vi "TSM SSC DAQmx Write (Digital Bool) Broadcast.vi"(0 "DAQ TSM in":T1, 1 "auto start(T)":bool=TRUE, 5 "Static State In":bool, 11 "error in":errorcluster) -> (4 "DAQ TSM Out":T1, 15 "error out":errorcluster)   [LabVIEW 2020]
doc: "Writes Static Digital State to a task that contains one or more digital output channels for all sites."
uses:
  Pin Map/TSM DAQmx Multi-Task.ctl
  <vilib>/NI_TestStand_SemiconductorModule/NI_TestStand_Semiconductor_Module.lvlibp/PinMap/PinQueryContext/MultiplePinMultipleSessionQueryContext/MultiplePinMultipleSessionQueryContext.lvclass
  Pin Map/SSC DAQmx.ctl
  <vilib>/DAQmx/write.llb/DAQmx Write (Digital 1D Bool NChan 1Samp 1Line).vi
  <vilib>/DAQmx/miscellaneous.llb/DAQmx Fill In Error Info.vi
  <resource>/objmgr/daqmx.rc
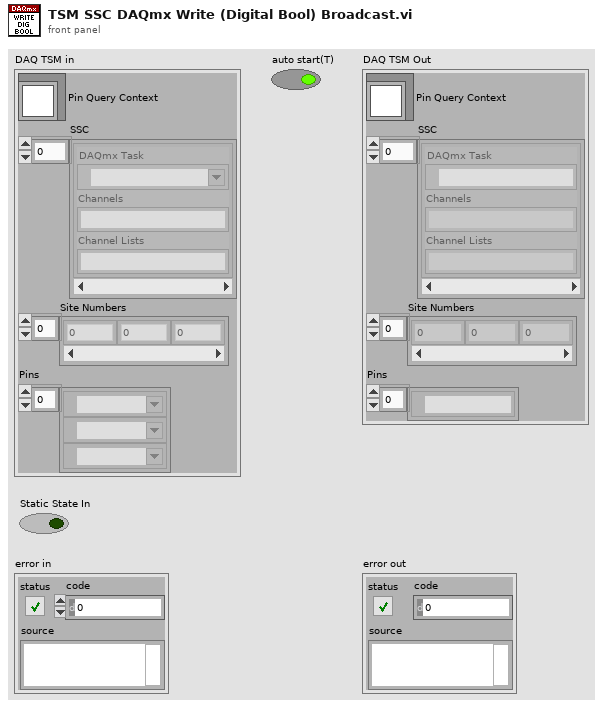
[diagram p1: front panel]
types:
  T1 = typedef "TSM DAQmx Multi-Task.ctl" = cluster{"Pin Query Context":refnum<class "MultiplePinMultipleSessionQueryContext.lvclass">, "SSC":T2[], "Site Numbers":i32[], "Pins":tag[]}
  T2 = typedef "SSC DAQmx.ctl" = cluster{"DAQmx Task ":refnum<k21>, "Channels":string, "Channel Lists":string}
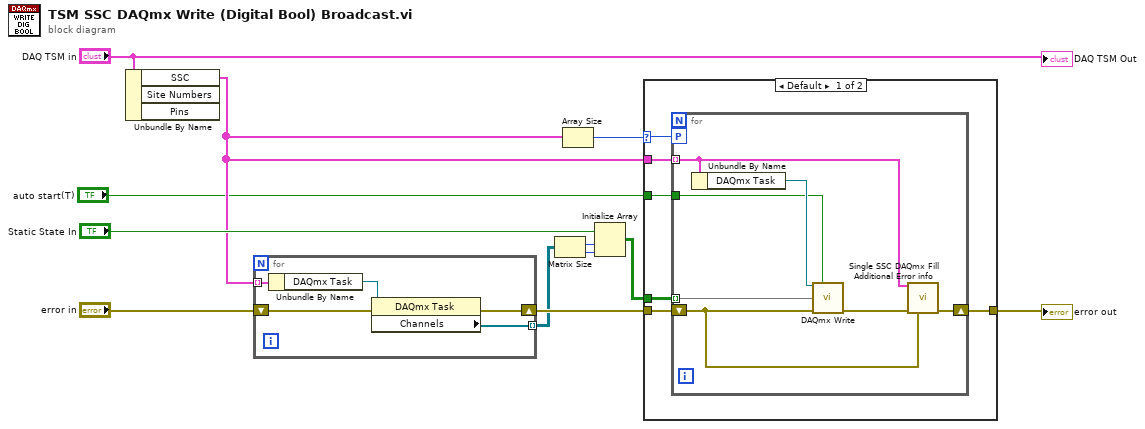
[diagram p0: block diagram]
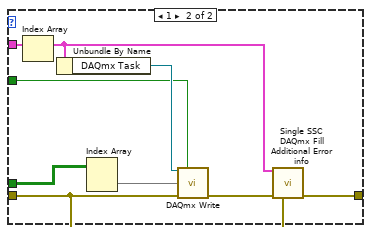
[diagram p2: hidden frame]
diagram:
  n1 = Unbundle By Name("DAQ TSM in") -> ("SSC"=w2:T2[])  [unwired: 2 out]
  n2 = for {
    shift-right: [w16] -> w8
    shift-left: "error in" -> [w17]
    tunnel: [w14] -> w5 mode=indexing
    tunnel: w2 -> [w13] mode=indexing
    n3 = Unbundle By Name(w13) -> ("DAQmx Task"=w15:refnum<k21>)
    n4 = property class="DAQmx Task"(reference=w15, error in=w17) -> (error out=w16:errorcluster, "Channels"=w14:refnum<k21>[])  [unwired: 1 out]
  }
  n5 = Matrix Size(0:w5) -> (1:w4:i32, 2:w3:i32)
  n6 = Array Size(array=w2) -> (size(s)=w9:i32)
  n7 = Initialize Array("Static State In", w4, w3) -> (w6:bool[][])
  n8 = case shown="Default" w9 {
    selector: w9 -> [w21 _]
    tunnel: [w23 w39] -> w10
    tunnel: w8 -> [w22 w38]
    tunnel: w2 -> [w20 w37]
    tunnel: w6 -> [w19 w33]
    tunnel: "auto start(T)" -> [w18 w31]
    frame Default {
      n9 = for {
        tunnel: w20 -> [w27] mode=indexing
        workers-P: w21 -> [_]
        shift-right: [w30] -> w23
        shift-left: w22 -> [w29]
        tunnel: w19 -> [w25] mode=indexing
        tunnel: w18 -> [w24]
        n10 = Unbundle By Name(w27) -> ("DAQmx Task"=w26:refnum<k21>)
        n11 = call-poly <vilib>:"DAQmx Write.vi"("task/channels in"=w26, "auto start"=w24, "data"=w25, "error in"=w29) -> ("error out"=w28:errorcluster)  [unwired: 9 in, 2 out]
        n12 = call "Single SSC DAQmx Fill Additional Error info.vi"("DAQmx SSC in"=w27, "error in"=w28, "previous error in"=w29) -> ("error out"=w30:errorcluster)  [unwired: 12 in]
      }
    }
    frame 1 {
      n13 = Index Array(array=w37) -> (element=w34:T2)  [unwired: 1 in]
      n14 = Unbundle By Name(w34) -> ("DAQmx Task"=w35:refnum<k21>)
      n15 = Index Array(array=w33) -> (element=w32:bool[])  [unwired: 2 in]
      n16 = call-poly <vilib>:"DAQmx Write.vi"("task/channels in"=w35, "auto start"=w31, "data"=w32, "error in"=w38) -> ("error out"=w36:errorcluster)  [unwired: 9 in, 2 out]
      n17 = call "Single SSC DAQmx Fill Additional Error info.vi"("DAQmx SSC in"=w34, "error in"=w36, "previous error in"=w38) -> ("error out"=w39:errorcluster)  [unwired: 12 in]
    }
  }
  "error out" <- w10
  "DAQ TSM Out" <- "DAQ TSM in"
